vi "fgt set sensor Calibration.vi"(8 "error in (no error)":errorcluster, 10 "calibration":T1=enum."H2O", 11 "sensorIndex":u32) -> (0 "error out":errorcluster)   [LabVIEW 2016, in "fgt_SDK.lvlib"]
doc: "Set used sensor internal calibration table. Function is only available for specific sensors such as the flow-unit M accepting H2O and IPA"
uses:
  fgt_SDK.lvlib
  TypeDefs/fgt_SENSOR_CALIBRATION.ctl
  dlls/fgt_SDK_32.dll
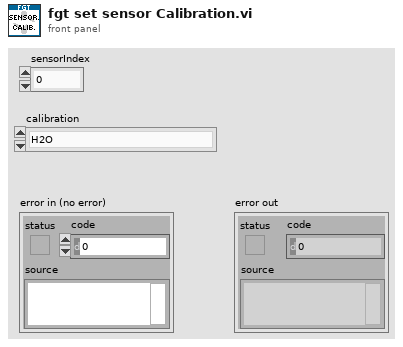
[diagram p1: front panel]
types:
  T1 = typedef "fgt_SDK.lvlib/fgt_SENSOR_CALIBRATION.ctl" = enum16{"None", "H2O", "IPA", "HFE", "FC40", "OIL"}
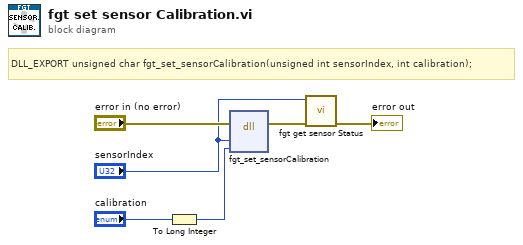
[diagram p0: block diagram]
diagram:
  # "DLL_EXPORT unsigned char fgt_set_sensorCalibration(unsigned int sensorIndex, int calibration);"
  n1 = To Long Integer(number="calibration") -> (32bit integer=w2:i32)
  n2 = dll-call lib="PTH2Zabs D\nMes DocumentsDéveloppementFluigentSDKsfgt-sdk-labviewdllsfgt_SDK_*.*" fn="fgt_set_sensorCalibration"(error in="error in (no error)", "sensorIndex"="sensorIndex", "calibration"=w2) -> (error out=w4:errorcluster)  [unwired: 5 in, 1 out]
  n3 = call "fgt get sensor Status.vi"("error in (no error)"=w4, "pressureIndex"="sensorIndex") -> ("error out"=→"error out":errorcluster)  [unwired: 9 in]
